vi "SE_HV200.ProcCases.vi"(0 "i ref in":refnum<vi>, 1 "selector":string, 2 "Data":T1, 3 "call cluster":T2={"Object"="", "Selector"="", "CallType"=enum."synchronous", "Async Object"="", "Async Selector"="", "Data Descriptor"="", "Data"=[], "Error #"=0, "Expire"=0}, 5 "error in (no error)":errorcluster) -> (14 "i ref out":refnum<vi>, 17 "answer cluster":T2={"Object"="", "Selector"="", "CallType"=enum."synchronous", "Async Object"="", "Async Selector"="", "Data Descriptor"="", "Data"=[], "Error #"=0, "Expire"=0}, 19 "error out":errorcluster)   [LabVIEW 2014, in "SE_HV200.lvlib"]
doc: "This method is called by a process from within the default case in the event loop. The methods of a class that are linked to events will be called from THIS method. Add your code here."
uses:
  SE_HV200.lvlib
  CS_Core/BaseProcess/BaseProcess.lvlib
  CS_Core/CSSystem/CoreLib/CoreLib.lvlib
  CS_Core/CSSystem/CoreLib/CoreLib.string 2 byte array.vi
  CS_Core/CSSystem/CoreLib/CoreLib.byte array 2 double.vi
  CS_Core/CSSystem/CoreLib/CoreLib.byte array 2 int.vi
  CS_Core/CSSystem/CoreDefs/CoreDefs.call_type.ctl
  CS_Core/BaseProcess/BaseProcess.descriptor string definition.ctl
  CS_Core/CSSystem/CoreDefs/CoreDefs.rawDataType.ctl
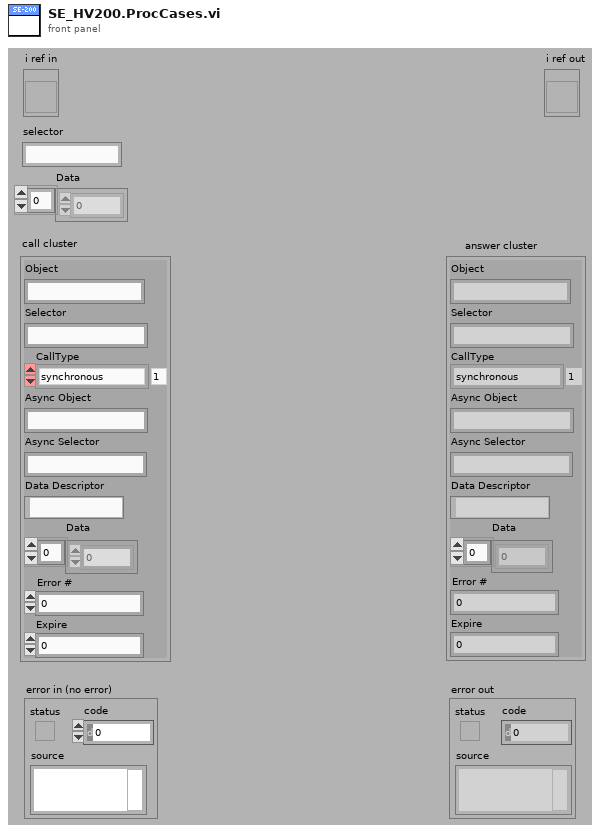
[diagram p1: front panel]
types:
  T1 = typedef "CoreDefs.rawDataType.ctl" = i8[]
  T2 = typedef "CoreDefs.call_type.ctl" = cluster{"Object":string, "Selector":string, "CallType":enum16{"simple", "synchronous", "asynchronous"}, "Async Object":string, "Async Selector":string, "Data Descriptor":T3, "Data":T1, "Error #":i32, "Expire":u32}
  T3 = typedef "BaseProcess.lvlib/BaseProcess.descriptor string definition.ctl" = string
  T4 = typedef "SE_HV200.lvlib/SE_HV200.i attribute.ctl" = cluster{"SetStatus":bool, "actVoltageID":i32, "VISA resource name in":refnum<visa-resource-name>, "Device name":string, "PSRange":i32, "nomVoltageID":i32, "actStatusID":i32, "NomVoltage":dbl[], "ActVoltage":dbl[], "DefaultChannel":i32}
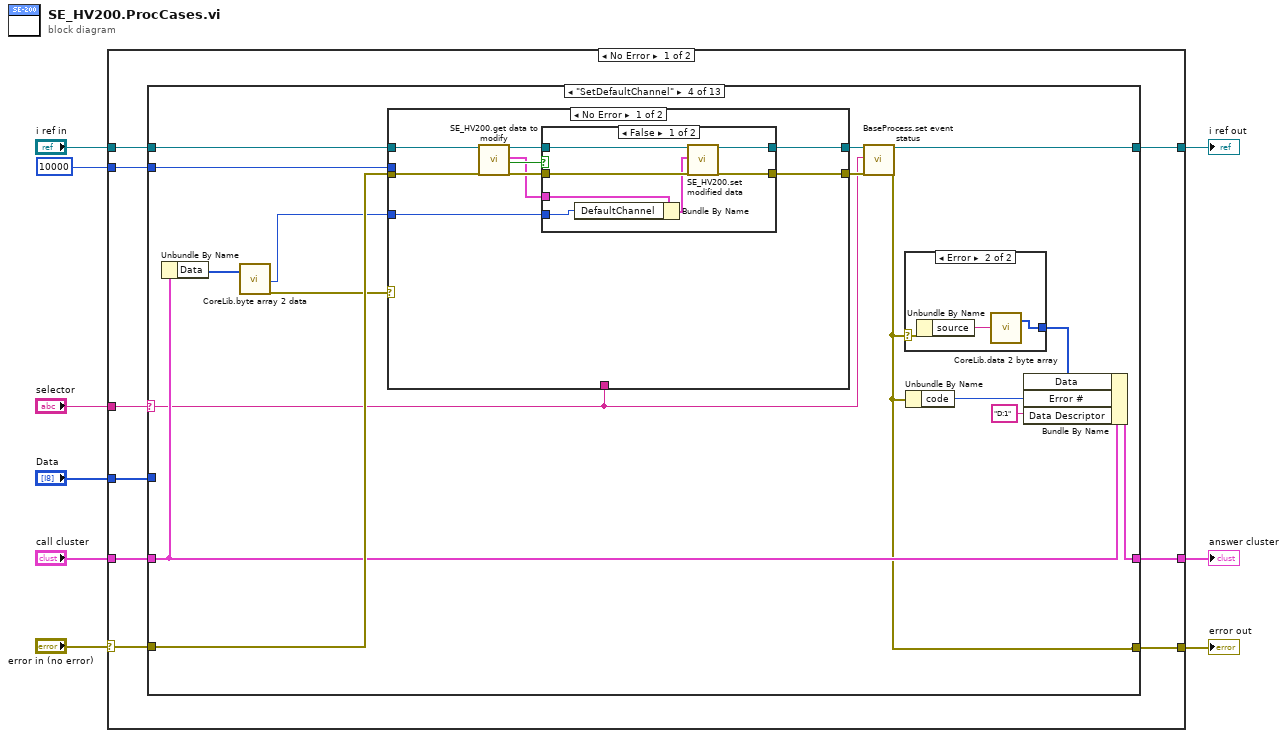
[diagram p0: block diagram]
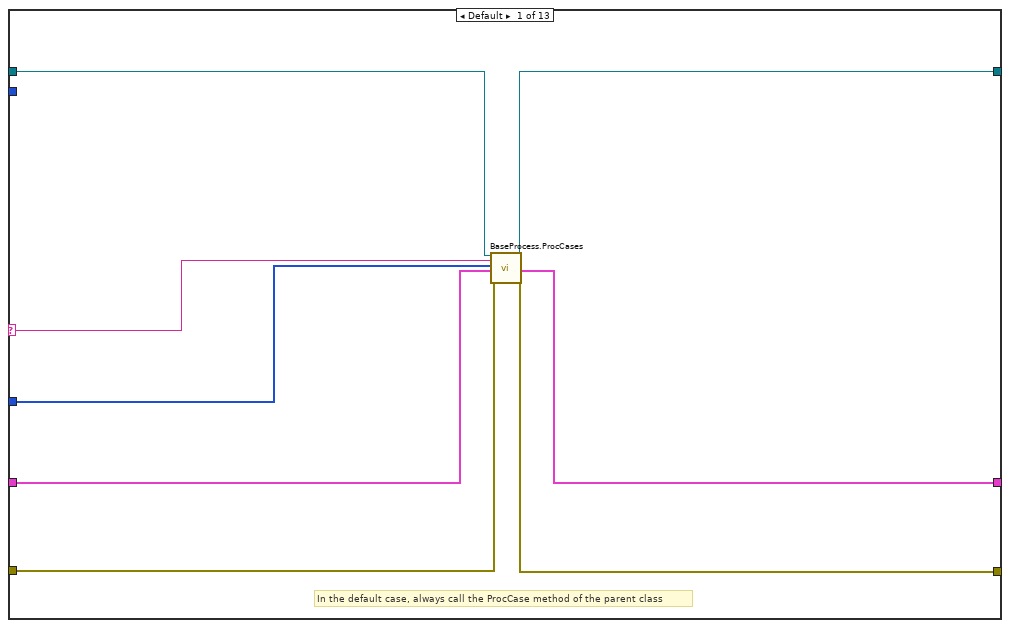
[diagram p2: hidden frame]
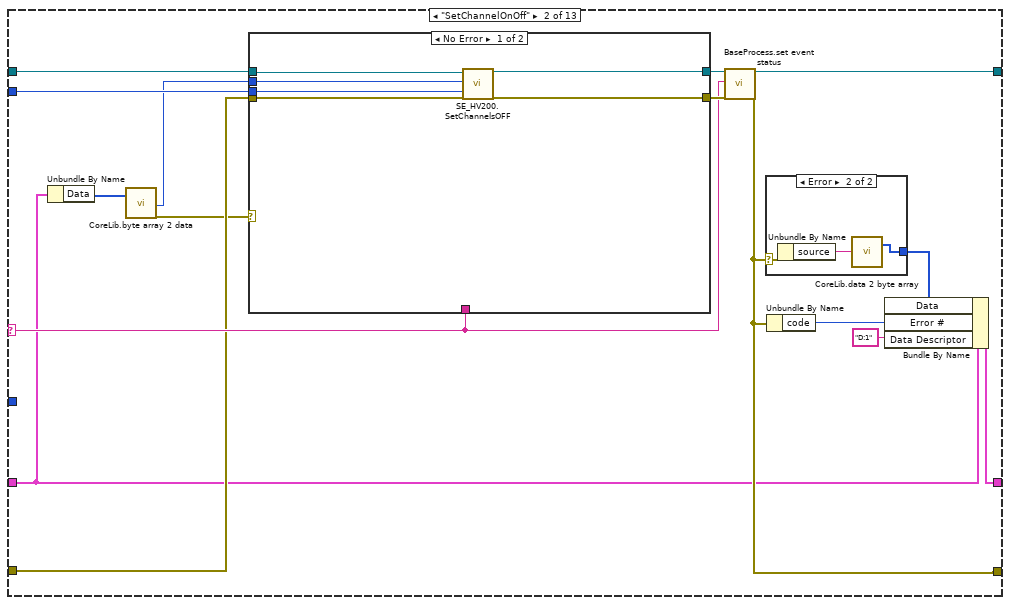
[diagram p3: hidden frame]
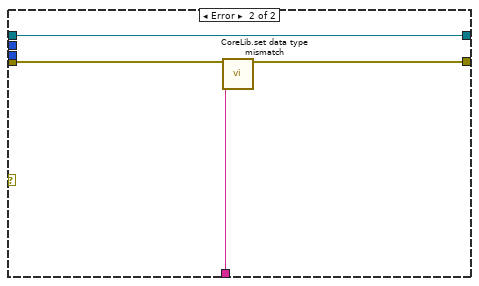
[diagram p5: hidden frame]
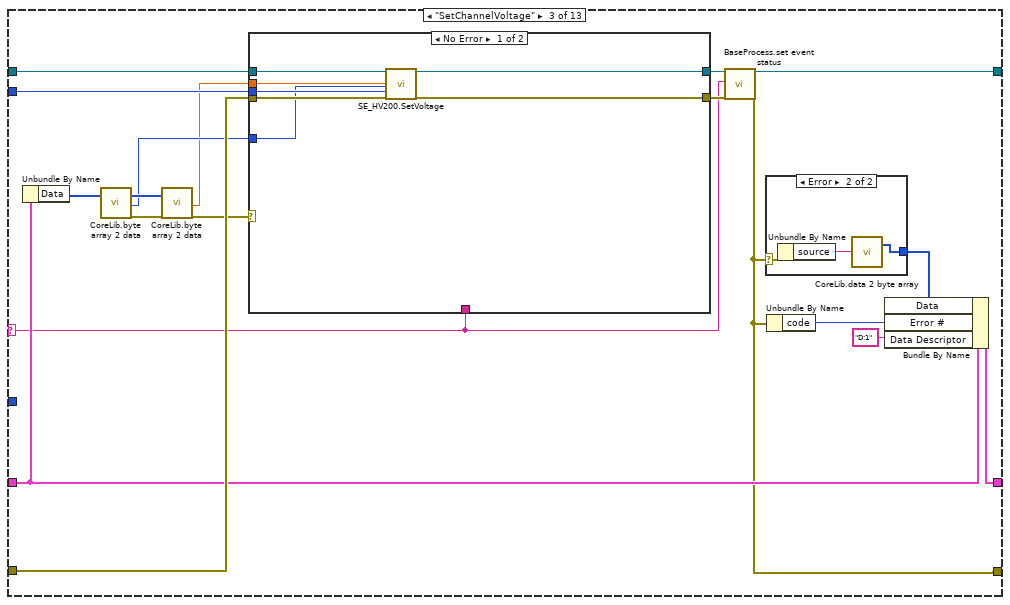
[diagram p6: hidden frame]
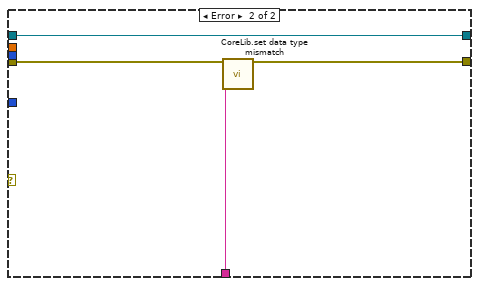
[diagram p8: hidden frame]
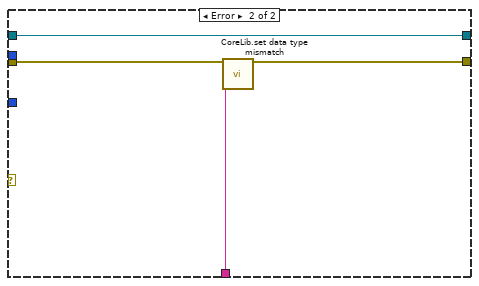
[diagram p11: hidden frame]
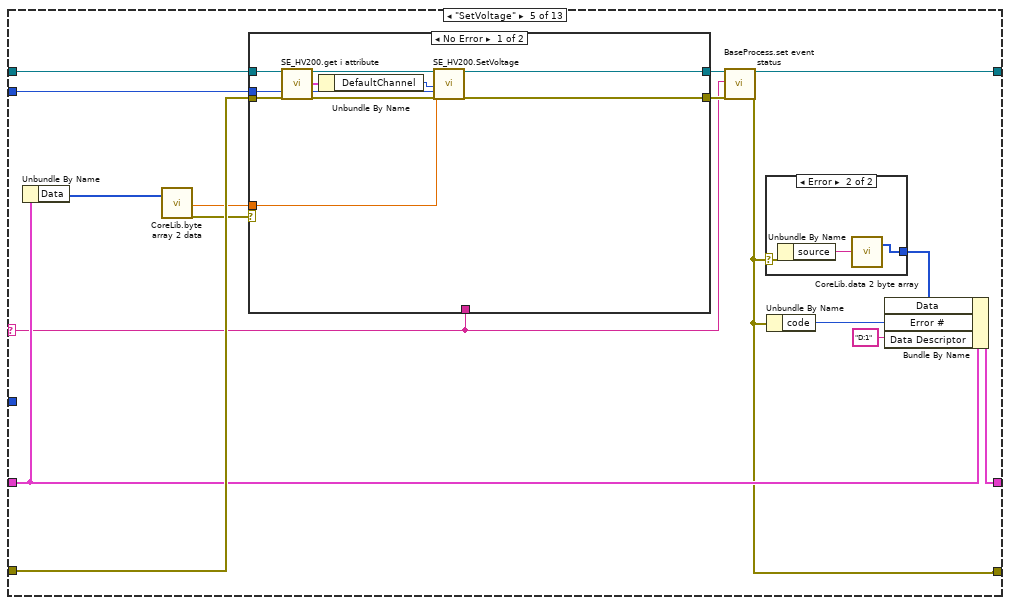
[diagram p12: hidden frame]
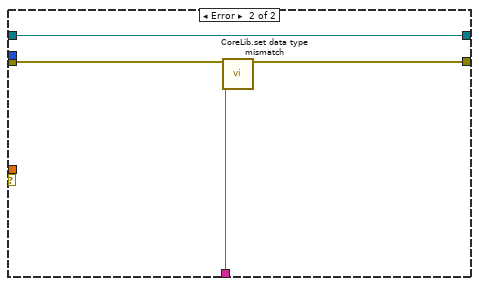
[diagram p14: hidden frame]
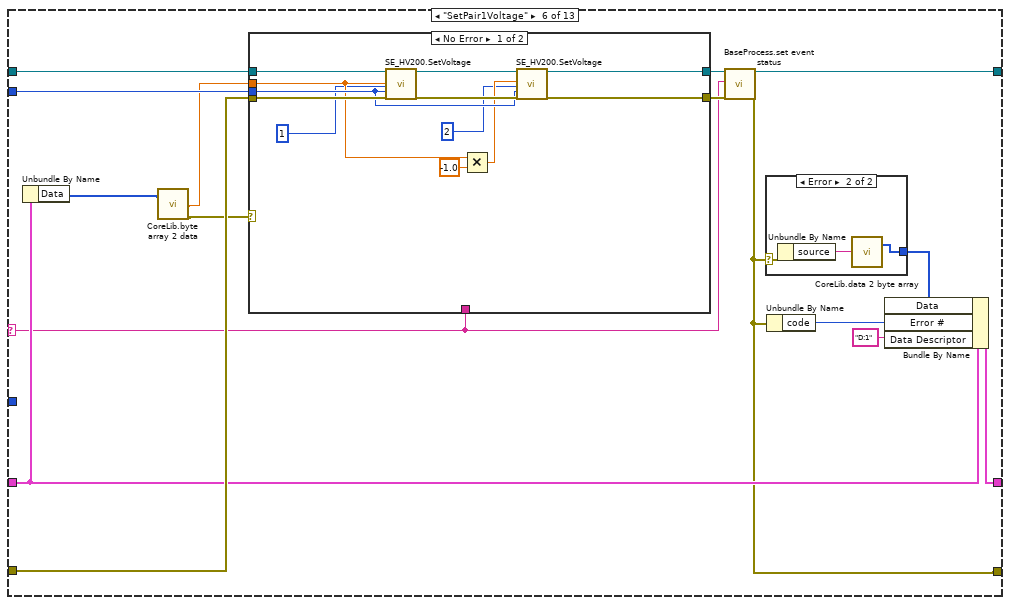
[diagram p15: hidden frame]
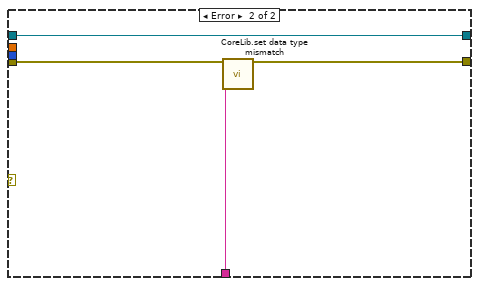
[diagram p17: hidden frame]
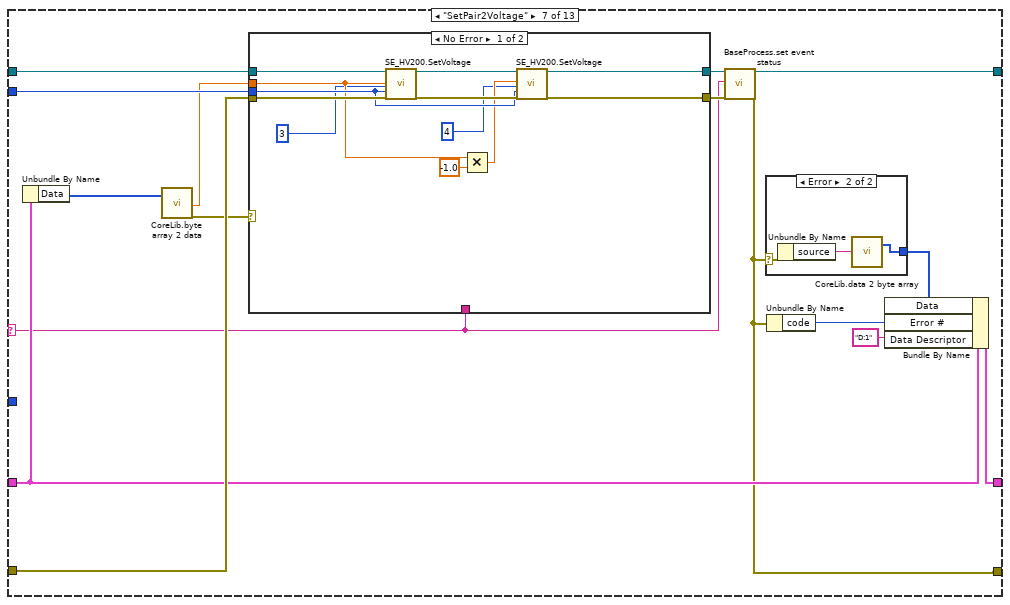
[diagram p18: hidden frame]
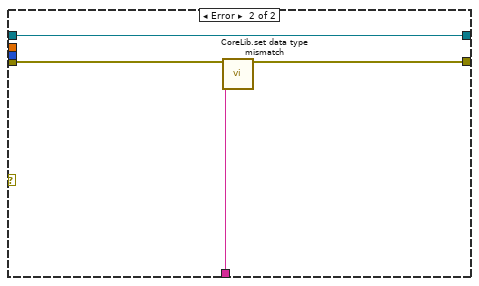
[diagram p20: hidden frame]
diagram:
  n1 = case shown="No Error" "error in (no error)" {
    selector: "error in (no error)" -> [w10 w443]
    tunnel: "selector" -> [w18 _]
    tunnel: [w17 w444] -> w8
    tunnel: "call cluster" -> [w16 w444]
    tunnel: "i ref in" -> [w15 w445]
    tunnel: [w14 w445] -> w5
    tunnel: [w13 w443] -> w4
    tunnel: 10000 -> [w12 _]
    tunnel: "Data" -> [w11 _]
    frame No Error {
      n2 = case shown="\"SetDefaultChannel\"" w18 {
        selector: w18 -> [w20 w35 w65 w95 w136 w169 w204 w239 w274 w309 w344 w379 w414]
        tunnel: w11 -> [w21 _ _ _ _ _ _ _ _ _ _ _ _]
        tunnel: w15 -> [w19 w42 w74 w104 w145 w178 w213 w248 w283 w318 w353 w388 w423]
        tunnel: [w26 w34 w64 w94 w135 w168 w203 w238 w273 w308 w343 w378 w413] -> w14
        tunnel: w16 -> [w22 w28 w71 w101 w142 w175 w210 w245 w280 w315 w350 w385 w420]
        tunnel: [w23 w40 w70 w100 w141 w174 w209 w244 w279 w314 w349 w384 w419] -> w17
        tunnel: w10 -> [w25 w31 w73 w103 w144 w177 w212 w247 w282 w317 w352 w387 w422]
        tunnel: [w24 w36 w66 w96 w137 w170 w205 w240 w275 w310 w345 w380 w415] -> w13
        tunnel: w12 -> [_ w32 w62 w92 w133 w166 w201 w236 w271 w306 w341 w376 w411]
        frame Default {
          # "In the default case, always call the ProcCase method of the parent class"
          n3 = call "BaseProcess.ProcCases.vi"("i ref in"=w19, "selector"=w20, "Data"=w21, "call cluster"=w22, "error in (no error)"=w25) -> ("i ref out"=w26:refnum<vi>, "answer cluster"=w23:T2, "error out"=w24:errorcluster)  [unwired: 12 in]
        }
        frame "SetChannelOnOff" {
          n4 = Unbundle By Name(w28) -> ("Data"=w30:T1)
          n5 = call-poly "CoreLib.byte array 2 data.vi"("byteArray"=w30) -> ("i32"=w27:i32, "error out"=w29:errorcluster)  [unwired: 16 in, 1 out]
          n6 = case shown="No Error" w29 {
            tunnel: [w49 w55] -> w38
            tunnel: w42 -> [w50 w55]
            tunnel: w31 -> [w47 w54]
            tunnel: [w51 w53] -> w37
            tunnel: w35 -> [_ w52]
            tunnel: w32 -> [w48 _]
            tunnel: w27 -> [w46 _]
            frame No Error {
              n7 = call "SE_HV200.SetChannelsOFF.vi"("i ref in"=w50, "Channel"=w46, "Time out"=w48, "error in (no error)"=w47) -> ("i ref out"=w49:refnum<vi>, "error out"=w51:errorcluster)  [unwired: 13 in, 1 out]
            }
            frame Error {
              n8 = call "CoreLib.set data type mismatch.vi"("error in (no error)"=w54, "error source"=w52) -> ("error out"=w53:errorcluster)  [unwired: 17 in]
            }
          }
          n9 = call "BaseProcess.set event status.vi"("i ref in"=w38, "EventStatus"=w35, "error in (no error)"=w37) -> ("i ref out"=w34:refnum<vi>, "error out"=w36:errorcluster)  [unwired: 14 in, 1 out]
          n10 = case shown="Error" w36 {
            selector: w36 -> [_ w45]
            tunnel: [_ w43] -> w39
            frame No Error {
            }
            frame Error {
              n11 = Unbundle By Name(w45) -> ("source"=w44:string)
              n12 = call-poly "CoreLib.data 2 byte array.vi"("string"=w44) -> ("byteArray out"=w43:T1)  [unwired: 18 in]
            }
          }
          n13 = Unbundle By Name(w36) -> ("code"=w41:i32)
          n14 = Bundle By Name(cluster=w28, "Data"=w39, "Error #"=w41, "Data Descriptor"="D:1") -> (w40:T2)
        }
        frame "SetChannelVoltage" {
          n15 = Unbundle By Name(w71) -> ("Data"=w61:T1)
          n16 = call-poly "CoreLib.byte array 2 data.vi"("byteArray"=w61) -> ("byteArray out"=w60:T1, "i32"=w57:i32, "error out"=w58:errorcluster)  [unwired: 16 in]
          n17 = call-poly "CoreLib.byte array 2 data.vi"("byteArray"=w60, "error in (no error)"=w58) -> ("d64"=w56:dbl, "error out"=w59:errorcluster)  [unwired: 15 in, 1 out]
          n18 = case shown="No Error" w59 {
            tunnel: [w79 w88] -> w68
            tunnel: w74 -> [w83 w88]
            tunnel: w73 -> [w84 w87]
            tunnel: [w80 w86] -> w67
            tunnel: w65 -> [_ w85]
            tunnel: w56 -> [w81 _]
            tunnel: w62 -> [w82 _]
            tunnel: w57 -> [w78 _]
            frame No Error {
              n19 = call "SE_HV200.SetVoltage.vi"("i ref in"=w83, "Set Voltage"=w81, "Channel"=w78, "Time out"=w82, "error in (no error)"=w84) -> ("i ref out"=w79:refnum<vi>, "error out"=w80:errorcluster)  [unwired: 12 in, 1 out]
            }
            frame Error {
              n20 = call "CoreLib.set data type mismatch.vi"("error in (no error)"=w87, "error source"=w85) -> ("error out"=w86:errorcluster)  [unwired: 17 in]
            }
          }
          n21 = call "BaseProcess.set event status.vi"("i ref in"=w68, "EventStatus"=w65, "error in (no error)"=w67) -> ("i ref out"=w64:refnum<vi>, "error out"=w66:errorcluster)  [unwired: 14 in, 1 out]
          n22 = case shown="Error" w66 {
            selector: w66 -> [_ w77]
            tunnel: [_ w75] -> w69
            frame No Error {
            }
            frame Error {
              n23 = Unbundle By Name(w77) -> ("source"=w76:string)
              n24 = call-poly "CoreLib.data 2 byte array.vi"("string"=w76) -> ("byteArray out"=w75:T1)  [unwired: 18 in]
            }
          }
          n25 = Unbundle By Name(w66) -> ("code"=w72:i32)
          n26 = Bundle By Name(cluster=w71, "Data"=w69, "Error #"=w72, "Data Descriptor"="D:1") -> (w70:T2)
        }
        frame "SetDefaultChannel" {
          n27 = Unbundle By Name(w101) -> ("Data"=w91:T1)
          n28 = call-poly "CoreLib.byte array 2 data.vi"("byteArray"=w91) -> ("i32"=w90:i32, "error out"=w89:errorcluster)  [unwired: 16 in, 1 out]
          n29 = case shown="No Error" w89 {
            tunnel: [w112 w129] -> w98
            tunnel: w104 -> [w116 w129]
            tunnel: w103 -> [w115 w128]
            tunnel: [w111 w127] -> w97
            tunnel: w95 -> [_ w126]
            tunnel: w92 -> [_ _]
            tunnel: w90 -> [w108 _]
            frame No Error {
              n30 = call "SE_HV200.get data to modify.vi"("i ref in"=w116, "error in (no error)"=w115) -> ("i ref out"=w114:refnum<vi>, "i attribute"=w109:T4, "timed out"=w110:bool, "error out"=w113:errorcluster)  [unwired: 14 in]
              n31 = case shown="False" w110 {
                tunnel: w114 -> [w123 w124]
                tunnel: w113 -> [w122 w125]
                tunnel: [w121 w124] -> w112
                tunnel: [w120 w125] -> w111
                tunnel: w109 -> [w119 _]
                tunnel: w108 -> [w117 _]
                frame False {
                  n32 = Bundle By Name(cluster=w119, "DefaultChannel"=w117) -> (w118:T4)
                  n33 = call "SE_HV200.set modified data.vi"("i ref in"=w123, "i attribute"=w118, "error in (no error)"=w122) -> ("i ref out"=w121:refnum<vi>, "error out"=w120:errorcluster)  [unwired: 15 in]
                }
                frame True {
                }
              }
            }
            frame Error {
              n34 = call "CoreLib.set data type mismatch.vi"("error in (no error)"=w128, "error source"=w126) -> ("error out"=w127:errorcluster)  [unwired: 17 in]
            }
          }
          n35 = call "BaseProcess.set event status.vi"("i ref in"=w98, "EventStatus"=w95, "error in (no error)"=w97) -> ("i ref out"=w94:refnum<vi>, "error out"=w96:errorcluster)  [unwired: 14 in, 1 out]
          n36 = case shown="Error" w96 {
            selector: w96 -> [_ w107]
            tunnel: [_ w105] -> w99
            frame No Error {
            }
            frame Error {
              n37 = Unbundle By Name(w107) -> ("source"=w106:string)
              n38 = call-poly "CoreLib.data 2 byte array.vi"("string"=w106) -> ("byteArray out"=w105:T1)  [unwired: 18 in]
            }
          }
          n39 = Unbundle By Name(w96) -> ("code"=w102:i32)
          n40 = Bundle By Name(cluster=w101, "Data"=w99, "Error #"=w102, "Data Descriptor"="D:1") -> (w100:T2)
        }
        frame "SetVoltage" {
          n41 = Unbundle By Name(w142) -> ("Data"=w130:T1)
          n42 = call-poly "CoreLib.byte array 2 data.vi"("byteArray"=w130) -> ("d64"=w131:dbl, "error out"=w132:errorcluster)  [unwired: 16 in, 1 out]
          n43 = case shown="No Error" w132 {
            tunnel: [w155 w162] -> w139
            tunnel: w145 -> [w154 w162]
            tunnel: w144 -> [w151 w161]
            tunnel: [w156 w160] -> w138
            tunnel: w136 -> [_ w159]
            tunnel: w131 -> [w157 _]
            tunnel: w133 -> [w158 _]
            frame No Error {
              n44 = call "SE_HV200.get i attribute.vi"("i ref in"=w154, "error in (no error)"=w151) -> ("i ref out"=w153:refnum<vi>, "i attribute"=w150:T4, "error out"=w152:errorcluster)  [unwired: 15 in]
              n45 = Unbundle By Name(w150) -> ("DefaultChannel"=w149:i32)
              n46 = call "SE_HV200.SetVoltage.vi"("i ref in"=w153, "Set Voltage"=w157, "Channel"=w149, "Time out"=w158, "error in (no error)"=w152) -> ("i ref out"=w155:refnum<vi>, "error out"=w156:errorcluster)  [unwired: 12 in, 1 out]
            }
            frame Error {
              n47 = call "CoreLib.set data type mismatch.vi"("error in (no error)"=w161, "error source"=w159) -> ("error out"=w160:errorcluster)  [unwired: 17 in]
            }
          }
          n48 = call "BaseProcess.set event status.vi"("i ref in"=w139, "EventStatus"=w136, "error in (no error)"=w138) -> ("i ref out"=w135:refnum<vi>, "error out"=w137:errorcluster)  [unwired: 14 in, 1 out]
          n49 = case shown="Error" w137 {
            selector: w137 -> [_ w148]
            tunnel: [_ w146] -> w140
            frame No Error {
            }
            frame Error {
              n50 = Unbundle By Name(w148) -> ("source"=w147:string)
              n51 = call-poly "CoreLib.data 2 byte array.vi"("string"=w147) -> ("byteArray out"=w146:T1)  [unwired: 18 in]
            }
          }
          n52 = Unbundle By Name(w137) -> ("code"=w143:i32)
          n53 = Bundle By Name(cluster=w142, "Data"=w140, "Error #"=w143, "Data Descriptor"="D:1") -> (w141:T2)
        }
        frame "SetPair1Voltage" {
          n54 = Unbundle By Name(w175) -> ("Data"=w164:T1)
          n55 = call-poly "CoreLib.byte array 2 data.vi"("byteArray"=w164) -> ("d64"=w163:dbl, "error out"=w165:errorcluster)  [unwired: 16 in, 1 out]
          n56 = case shown="No Error" w165 {
            tunnel: [w188 w197] -> w172
            tunnel: w178 -> [w192 w197]
            tunnel: w177 -> [w193 w196]
            tunnel: [w190 w195] -> w171
            tunnel: w169 -> [_ w194]
            tunnel: w163 -> [w185 _]
            tunnel: w166 -> [w187 _]
            frame No Error {
              n57 = call "SE_HV200.SetVoltage.vi"("i ref in"=w192, "Set Voltage"=w185, "Channel"=i16 1, "Time out"=w187, "error in (no error)"=w193) -> ("i ref out"=w189:refnum<vi>, "error out"=w191:errorcluster)  [unwired: 12 in, 1 out]
              n58 = Multiply(x=w185, y=-1.0) -> (x*y=w184:dbl)
              n59 = call "SE_HV200.SetVoltage.vi"("i ref in"=w189, "Set Voltage"=w184, "Channel"=i16 2, "Time out"=w187, "error in (no error)"=w191) -> ("i ref out"=w188:refnum<vi>, "error out"=w190:errorcluster)  [unwired: 12 in, 1 out]
            }
            frame Error {
              n60 = call "CoreLib.set data type mismatch.vi"("error in (no error)"=w196, "error source"=w194) -> ("error out"=w195:errorcluster)  [unwired: 17 in]
            }
          }
          n61 = call "BaseProcess.set event status.vi"("i ref in"=w172, "EventStatus"=w169, "error in (no error)"=w171) -> ("i ref out"=w168:refnum<vi>, "error out"=w170:errorcluster)  [unwired: 14 in, 1 out]
          n62 = case shown="Error" w170 {
            selector: w170 -> [_ w181]
            tunnel: [_ w179] -> w173
            frame No Error {
            }
            frame Error {
              n63 = Unbundle By Name(w181) -> ("source"=w180:string)
              n64 = call-poly "CoreLib.data 2 byte array.vi"("string"=w180) -> ("byteArray out"=w179:T1)  [unwired: 18 in]
            }
          }
          n65 = Unbundle By Name(w170) -> ("code"=w176:i32)
          n66 = Bundle By Name(cluster=w175, "Data"=w173, "Error #"=w176, "Data Descriptor"="D:1") -> (w174:T2)
        }
        frame "SetPair2Voltage" {
          n67 = Unbundle By Name(w210) -> ("Data"=w199:T1)
          n68 = call-poly "CoreLib.byte array 2 data.vi"("byteArray"=w199) -> ("d64"=w198:dbl, "error out"=w200:errorcluster)  [unwired: 16 in, 1 out]
          n69 = case shown="No Error" w200 {
            tunnel: [w223 w232] -> w207
            tunnel: w213 -> [w227 w232]
            tunnel: w212 -> [w228 w231]
            tunnel: [w225 w230] -> w206
            tunnel: w204 -> [_ w229]
            tunnel: w198 -> [w220 _]
            tunnel: w201 -> [w222 _]
            frame No Error {
              n70 = call "SE_HV200.SetVoltage.vi"("i ref in"=w227, "Set Voltage"=w220, "Channel"=i16 3, "Time out"=w222, "error in (no error)"=w228) -> ("i ref out"=w224:refnum<vi>, "error out"=w226:errorcluster)  [unwired: 12 in, 1 out]
              n71 = Multiply(x=w220, y=-1.0) -> (x*y=w219:dbl)
              n72 = call "SE_HV200.SetVoltage.vi"("i ref in"=w224, "Set Voltage"=w219, "Channel"=i16 4, "Time out"=w222, "error in (no error)"=w226) -> ("i ref out"=w223:refnum<vi>, "error out"=w225:errorcluster)  [unwired: 12 in, 1 out]
            }
            frame Error {
              n73 = call "CoreLib.set data type mismatch.vi"("error in (no error)"=w231, "error source"=w229) -> ("error out"=w230:errorcluster)  [unwired: 17 in]
            }
          }
          n74 = call "BaseProcess.set event status.vi"("i ref in"=w207, "EventStatus"=w204, "error in (no error)"=w206) -> ("i ref out"=w203:refnum<vi>, "error out"=w205:errorcluster)  [unwired: 14 in, 1 out]
          n75 = case shown="Error" w205 {
            selector: w205 -> [_ w216]
            tunnel: [_ w214] -> w208
            frame No Error {
            }
            frame Error {
              n76 = Unbundle By Name(w216) -> ("source"=w215:string)
              n77 = call-poly "CoreLib.data 2 byte array.vi"("string"=w215) -> ("byteArray out"=w214:T1)  [unwired: 18 in]
            }
          }
          n78 = Unbundle By Name(w205) -> ("code"=w211:i32)
          n79 = Bundle By Name(cluster=w210, "Data"=w208, "Error #"=w211, "Data Descriptor"="D:1") -> (w209:T2)
        }
        frame "SetPair3Voltage" {
          n80 = Unbundle By Name(w245) -> ("Data"=w234:T1)
          n81 = call-poly "CoreLib.byte array 2 data.vi"("byteArray"=w234) -> ("d64"=w233:dbl, "error out"=w235:errorcluster)  [unwired: 16 in, 1 out]
          n82 = case shown="No Error" w235 {
            tunnel: [w258 w267] -> w242
            tunnel: w248 -> [w262 w267]
            tunnel: w247 -> [w263 w266]
            tunnel: [w260 w265] -> w241
            tunnel: w239 -> [_ w264]
            tunnel: w233 -> [w255 _]
            tunnel: w236 -> [w257 _]
            frame No Error {
              n83 = call "SE_HV200.SetVoltage.vi"("i ref in"=w262, "Set Voltage"=w255, "Channel"=i16 5, "Time out"=w257, "error in (no error)"=w263) -> ("i ref out"=w259:refnum<vi>, "error out"=w261:errorcluster)  [unwired: 12 in, 1 out]
              n84 = Multiply(x=w255, y=-1.0) -> (x*y=w254:dbl)
              n85 = call "SE_HV200.SetVoltage.vi"("i ref in"=w259, "Set Voltage"=w254, "Channel"=i16 6, "Time out"=w257, "error in (no error)"=w261) -> ("i ref out"=w258:refnum<vi>, "error out"=w260:errorcluster)  [unwired: 12 in, 1 out]
            }
            frame Error {
              n86 = call "CoreLib.set data type mismatch.vi"("error in (no error)"=w266, "error source"=w264) -> ("error out"=w265:errorcluster)  [unwired: 17 in]
            }
          }
          n87 = call "BaseProcess.set event status.vi"("i ref in"=w242, "EventStatus"=w239, "error in (no error)"=w241) -> ("i ref out"=w238:refnum<vi>, "error out"=w240:errorcluster)  [unwired: 14 in, 1 out]
          n88 = case shown="Error" w240 {
            selector: w240 -> [_ w251]
            tunnel: [_ w249] -> w243
            frame No Error {
            }
            frame Error {
              n89 = Unbundle By Name(w251) -> ("source"=w250:string)
              n90 = call-poly "CoreLib.data 2 byte array.vi"("string"=w250) -> ("byteArray out"=w249:T1)  [unwired: 18 in]
            }
          }
          n91 = Unbundle By Name(w240) -> ("code"=w246:i32)
          n92 = Bundle By Name(cluster=w245, "Data"=w243, "Error #"=w246, "Data Descriptor"="D:1") -> (w244:T2)
        }
        frame "SetPair4Voltage" {
          n93 = Unbundle By Name(w280) -> ("Data"=w269:T1)
          n94 = call-poly "CoreLib.byte array 2 data.vi"("byteArray"=w269) -> ("d64"=w268:dbl, "error out"=w270:errorcluster)  [unwired: 16 in, 1 out]
          n95 = case shown="No Error" w270 {
            tunnel: [w293 w302] -> w277
            tunnel: w283 -> [w297 w302]
            tunnel: w282 -> [w298 w301]
            tunnel: [w295 w300] -> w276
            tunnel: w274 -> [_ w299]
            tunnel: w268 -> [w290 _]
            tunnel: w271 -> [w292 _]
            frame No Error {
              n96 = call "SE_HV200.SetVoltage.vi"("i ref in"=w297, "Set Voltage"=w290, "Channel"=i16 7, "Time out"=w292, "error in (no error)"=w298) -> ("i ref out"=w294:refnum<vi>, "error out"=w296:errorcluster)  [unwired: 12 in, 1 out]
              n97 = Multiply(x=w290, y=-1.0) -> (x*y=w289:dbl)
              n98 = call "SE_HV200.SetVoltage.vi"("i ref in"=w294, "Set Voltage"=w289, "Channel"=i16 8, "Time out"=w292, "error in (no error)"=w296) -> ("i ref out"=w293:refnum<vi>, "error out"=w295:errorcluster)  [unwired: 12 in, 1 out]
            }
            frame Error {
              n99 = call "CoreLib.set data type mismatch.vi"("error in (no error)"=w301, "error source"=w299) -> ("error out"=w300:errorcluster)  [unwired: 17 in]
            }
          }
          n100 = call "BaseProcess.set event status.vi"("i ref in"=w277, "EventStatus"=w274, "error in (no error)"=w276) -> ("i ref out"=w273:refnum<vi>, "error out"=w275:errorcluster)  [unwired: 14 in, 1 out]
          n101 = case shown="Error" w275 {
            selector: w275 -> [_ w286]
            tunnel: [_ w284] -> w278
            frame No Error {
            }
            frame Error {
              n102 = Unbundle By Name(w286) -> ("source"=w285:string)
              n103 = call-poly "CoreLib.data 2 byte array.vi"("string"=w285) -> ("byteArray out"=w284:T1)  [unwired: 18 in]
            }
          }
          n104 = Unbundle By Name(w275) -> ("code"=w281:i32)
          n105 = Bundle By Name(cluster=w280, "Data"=w278, "Error #"=w281, "Data Descriptor"="D:1") -> (w279:T2)
        }
        frame "SetPair5Voltage" {
          n106 = Unbundle By Name(w315) -> ("Data"=w304:T1)
          n107 = call-poly "CoreLib.byte array 2 data.vi"("byteArray"=w304) -> ("d64"=w303:dbl, "error out"=w305:errorcluster)  [unwired: 16 in, 1 out]
          n108 = case shown="No Error" w305 {
            tunnel: [w328 w337] -> w312
            tunnel: w318 -> [w332 w337]
            tunnel: w317 -> [w333 w336]
            tunnel: [w330 w335] -> w311
            tunnel: w309 -> [_ w334]
            tunnel: w303 -> [w325 _]
            tunnel: w306 -> [w327 _]
            frame No Error {
              n109 = call "SE_HV200.SetVoltage.vi"("i ref in"=w332, "Set Voltage"=w325, "Channel"=i16 9, "Time out"=w327, "error in (no error)"=w333) -> ("i ref out"=w329:refnum<vi>, "error out"=w331:errorcluster)  [unwired: 12 in, 1 out]
              n110 = Multiply(x=w325, y=-1.0) -> (x*y=w324:dbl)
              n111 = call "SE_HV200.SetVoltage.vi"("i ref in"=w329, "Set Voltage"=w324, "Channel"=i16 10, "Time out"=w327, "error in (no error)"=w331) -> ("i ref out"=w328:refnum<vi>, "error out"=w330:errorcluster)  [unwired: 12 in, 1 out]
            }
            frame Error {
              n112 = call "CoreLib.set data type mismatch.vi"("error in (no error)"=w336, "error source"=w334) -> ("error out"=w335:errorcluster)  [unwired: 17 in]
            }
          }
          n113 = call "BaseProcess.set event status.vi"("i ref in"=w312, "EventStatus"=w309, "error in (no error)"=w311) -> ("i ref out"=w308:refnum<vi>, "error out"=w310:errorcluster)  [unwired: 14 in, 1 out]
          n114 = case shown="Error" w310 {
            selector: w310 -> [_ w321]
            tunnel: [_ w319] -> w313
            frame No Error {
            }
            frame Error {
              n115 = Unbundle By Name(w321) -> ("source"=w320:string)
              n116 = call-poly "CoreLib.data 2 byte array.vi"("string"=w320) -> ("byteArray out"=w319:T1)  [unwired: 18 in]
            }
          }
          n117 = Unbundle By Name(w310) -> ("code"=w316:i32)
          n118 = Bundle By Name(cluster=w315, "Data"=w313, "Error #"=w316, "Data Descriptor"="D:1") -> (w314:T2)
        }
        frame "SetPair6Voltage" {
          n119 = Unbundle By Name(w350) -> ("Data"=w339:T1)
          n120 = call-poly "CoreLib.byte array 2 data.vi"("byteArray"=w339) -> ("d64"=w338:dbl, "error out"=w340:errorcluster)  [unwired: 16 in, 1 out]
          n121 = case shown="No Error" w340 {
            tunnel: [w363 w372] -> w347
            tunnel: w353 -> [w367 w372]
            tunnel: w352 -> [w368 w371]
            tunnel: [w365 w370] -> w346
            tunnel: w344 -> [_ w369]
            tunnel: w338 -> [w360 _]
            tunnel: w341 -> [w362 _]
            frame No Error {
              n122 = call "SE_HV200.SetVoltage.vi"("i ref in"=w367, "Set Voltage"=w360, "Channel"=i16 11, "Time out"=w362, "error in (no error)"=w368) -> ("i ref out"=w364:refnum<vi>, "error out"=w366:errorcluster)  [unwired: 12 in, 1 out]
              n123 = Multiply(x=w360, y=-1.0) -> (x*y=w359:dbl)
              n124 = call "SE_HV200.SetVoltage.vi"("i ref in"=w364, "Set Voltage"=w359, "Channel"=i16 12, "Time out"=w362, "error in (no error)"=w366) -> ("i ref out"=w363:refnum<vi>, "error out"=w365:errorcluster)  [unwired: 12 in, 1 out]
            }
            frame Error {
              n125 = call "CoreLib.set data type mismatch.vi"("error in (no error)"=w371, "error source"=w369) -> ("error out"=w370:errorcluster)  [unwired: 17 in]
            }
          }
          n126 = call "BaseProcess.set event status.vi"("i ref in"=w347, "EventStatus"=w344, "error in (no error)"=w346) -> ("i ref out"=w343:refnum<vi>, "error out"=w345:errorcluster)  [unwired: 14 in, 1 out]
          n127 = case shown="Error" w345 {
            selector: w345 -> [_ w356]
            tunnel: [_ w354] -> w348
            frame No Error {
            }
            frame Error {
              n128 = Unbundle By Name(w356) -> ("source"=w355:string)
              n129 = call-poly "CoreLib.data 2 byte array.vi"("string"=w355) -> ("byteArray out"=w354:T1)  [unwired: 18 in]
            }
          }
          n130 = Unbundle By Name(w345) -> ("code"=w351:i32)
          n131 = Bundle By Name(cluster=w350, "Data"=w348, "Error #"=w351, "Data Descriptor"="D:1") -> (w349:T2)
        }
        frame "SetPair7Voltage" {
          n132 = Unbundle By Name(w385) -> ("Data"=w374:T1)
          n133 = call-poly "CoreLib.byte array 2 data.vi"("byteArray"=w374) -> ("d64"=w373:dbl, "error out"=w375:errorcluster)  [unwired: 16 in, 1 out]
          n134 = case shown="No Error" w375 {
            tunnel: [w398 w407] -> w382
            tunnel: w388 -> [w402 w407]
            tunnel: w387 -> [w403 w406]
            tunnel: [w400 w405] -> w381
            tunnel: w379 -> [_ w404]
            tunnel: w373 -> [w395 _]
            tunnel: w376 -> [w397 _]
            frame No Error {
              n135 = call "SE_HV200.SetVoltage.vi"("i ref in"=w402, "Set Voltage"=w395, "Channel"=i16 13, "Time out"=w397, "error in (no error)"=w403) -> ("i ref out"=w399:refnum<vi>, "error out"=w401:errorcluster)  [unwired: 12 in, 1 out]
              n136 = Multiply(x=w395, y=-1.0) -> (x*y=w394:dbl)
              n137 = call "SE_HV200.SetVoltage.vi"("i ref in"=w399, "Set Voltage"=w394, "Channel"=i16 14, "Time out"=w397, "error in (no error)"=w401) -> ("i ref out"=w398:refnum<vi>, "error out"=w400:errorcluster)  [unwired: 12 in, 1 out]
            }
            frame Error {
              n138 = call "CoreLib.set data type mismatch.vi"("error in (no error)"=w406, "error source"=w404) -> ("error out"=w405:errorcluster)  [unwired: 17 in]
            }
          }
          n139 = call "BaseProcess.set event status.vi"("i ref in"=w382, "EventStatus"=w379, "error in (no error)"=w381) -> ("i ref out"=w378:refnum<vi>, "error out"=w380:errorcluster)  [unwired: 14 in, 1 out]
          n140 = case shown="Error" w380 {
            selector: w380 -> [_ w391]
            tunnel: [_ w389] -> w383
            frame No Error {
            }
            frame Error {
              n141 = Unbundle By Name(w391) -> ("source"=w390:string)
              n142 = call-poly "CoreLib.data 2 byte array.vi"("string"=w390) -> ("byteArray out"=w389:T1)  [unwired: 18 in]
            }
          }
          n143 = Unbundle By Name(w380) -> ("code"=w386:i32)
          n144 = Bundle By Name(cluster=w385, "Data"=w383, "Error #"=w386, "Data Descriptor"="D:1") -> (w384:T2)
        }
        frame "SetPair8Voltage" {
          n145 = Unbundle By Name(w420) -> ("Data"=w409:T1)
          n146 = call-poly "CoreLib.byte array 2 data.vi"("byteArray"=w409) -> ("d64"=w408:dbl, "error out"=w410:errorcluster)  [unwired: 16 in, 1 out]
          n147 = case shown="No Error" w410 {
            tunnel: [w433 w442] -> w417
            tunnel: w423 -> [w437 w442]
            tunnel: w422 -> [w438 w441]
            tunnel: [w435 w440] -> w416
            tunnel: w414 -> [_ w439]
            tunnel: w408 -> [w430 _]
            tunnel: w411 -> [w432 _]
            frame No Error {
              n148 = call "SE_HV200.SetVoltage.vi"("i ref in"=w437, "Set Voltage"=w430, "Channel"=i16 15, "Time out"=w432, "error in (no error)"=w438) -> ("i ref out"=w434:refnum<vi>, "error out"=w436:errorcluster)  [unwired: 12 in, 1 out]
              n149 = Multiply(x=w430, y=-1.0) -> (x*y=w429:dbl)
              n150 = call "SE_HV200.SetVoltage.vi"("i ref in"=w434, "Set Voltage"=w429, "Channel"=i16 16, "Time out"=w432, "error in (no error)"=w436) -> ("i ref out"=w433:refnum<vi>, "error out"=w435:errorcluster)  [unwired: 12 in, 1 out]
            }
            frame Error {
              n151 = call "CoreLib.set data type mismatch.vi"("error in (no error)"=w441, "error source"=w439) -> ("error out"=w440:errorcluster)  [unwired: 17 in]
            }
          }
          n152 = call "BaseProcess.set event status.vi"("i ref in"=w417, "EventStatus"=w414, "error in (no error)"=w416) -> ("i ref out"=w413:refnum<vi>, "error out"=w415:errorcluster)  [unwired: 14 in, 1 out]
          n153 = case shown="Error" w415 {
            selector: w415 -> [_ w426]
            tunnel: [_ w424] -> w418
            frame No Error {
            }
            frame Error {
              n154 = Unbundle By Name(w426) -> ("source"=w425:string)
              n155 = call-poly "CoreLib.data 2 byte array.vi"("string"=w425) -> ("byteArray out"=w424:T1)  [unwired: 18 in]
            }
          }
          n156 = Unbundle By Name(w415) -> ("code"=w421:i32)
          n157 = Bundle By Name(cluster=w420, "Data"=w418, "Error #"=w421, "Data Descriptor"="D:1") -> (w419:T2)
        }
      }
    }
    frame Error {
    }
  }
  "answer cluster" <- w8
  "i ref out" <- w5
  "error out" <- w4
